vi "Select Controls.vi"(10 "All Controls[]":refnum<vi>[](array[refnum])) -> (1 "OK?":bool, 2 "Listbox 2":i32[](listbox), 3 "Operation":T1, 4 "Create Properties 2":bool, 5 "isDynamic?":bool)   [LabVIEW 2018, in "DVR Accessor Library.lvlib"]
uses:
  DVR Accessor Library.lvlib
  TypeDef/Accessor Type.ctl
panel:
  in  "Create Properties":bool
  in  "Scope":enum32{"Item 0", "Item 1"}(radio)
  in  "Type":T1
  in  "Cancel":bool
  in  "OK":bool
  in  "Listbox":i32[](listbox)
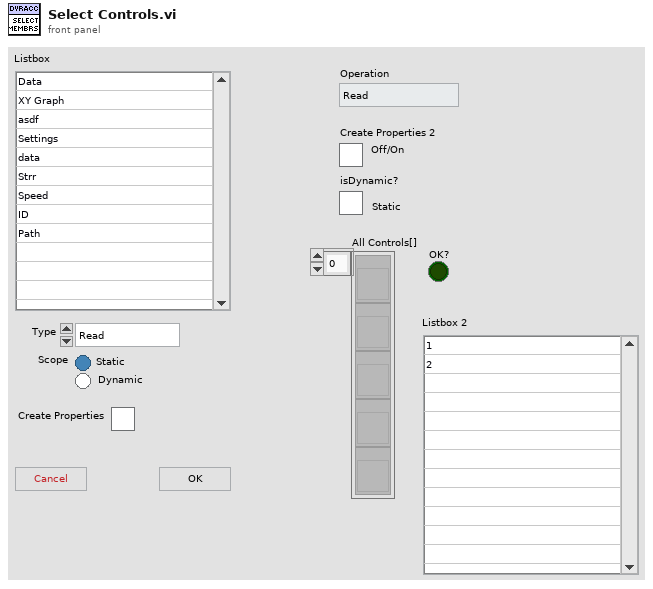
[diagram p1: front panel]
types:
  T1 = typedef "DVR Accessor Library.lvlib/Accessor Type.ctl" = enum16{"Read", "Read And Write", "Write"}
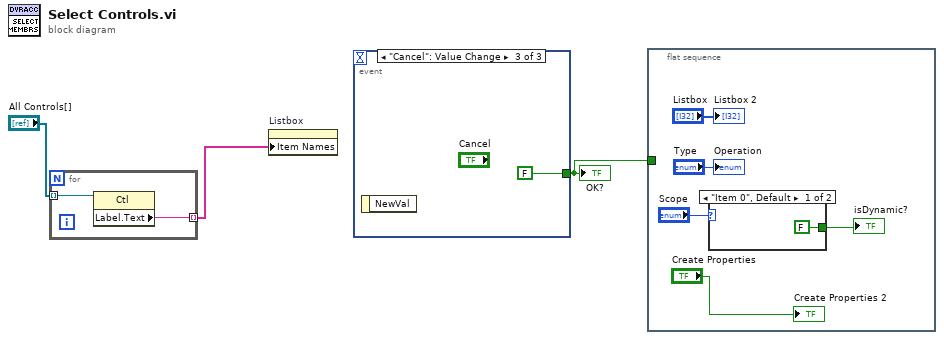
[diagram p0: block diagram]
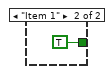
[diagram p2: hidden frame]
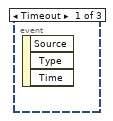
[diagram p3: hidden frame]
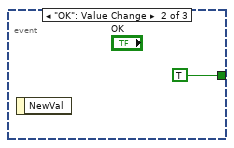
[diagram p4: hidden frame]
diagram:
  n1 = for {
    tunnel: "All Controls[]" -> [w5] mode=indexing
    tunnel: [w4] -> w1 mode=indexing
    n2 = property class="Ctl"(reference=w5) -> ("Label.Text"=w4:string)  [unwired: 1 in, 2 out]
  }
  n3 = property on="Listbox" class="LstBox (strict)"("Item Names"=w1) -> ()  [unwired: 2 in, 2 out]
  n4 = event shown="[2] \"Cancel\": Value Change" {
    selector: _ -> [_ _ _]
    dyn-events: _ -> [_ _ _]
    timeout: _ -> [_ _ _]
    tunnel: [_ TRUE FALSE] -> w3
    event Timeout {
      n5 = event-data() -> ()  [unwired: 1 in, 3 out]
    }
    event "OK": Value Change {
      n6 = event-data() -> ()  [unwired: 1 in, 1 out]
    }
    event "Cancel": Value Change {
      n7 = event-data() -> ()  [unwired: 1 in, 1 out]
    }
  }
  "OK?" <- w3
  n8 = flat-sequence {
    tunnel: w3 -> [_]
    frame #0 {
      n9 = case shown="\"Item 0\", Default" "Scope" {
        tunnel: [FALSE TRUE] -> w8
        frame "Item 0", Default {
        }
        frame "Item 1" {
        }
      }
      "isDynamic?" <- w8
      "Listbox 2" <- "Listbox"
      "Operation" <- "Type"
      "Create Properties 2" <- "Create Properties"
    }
  }
